vi "Describe Double Failure.vi"(1 "Expected":dbl, 2 "Got":dbl) -> (0 "Failure Description":string)   [LabVIEW 2013]
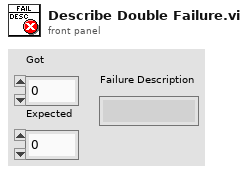
[diagram p1: front panel]
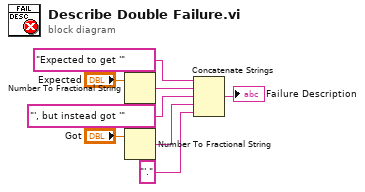
[diagram p0: block diagram]
diagram:
  n1 = Number To Fractional String(number="Expected") -> (F-format string=w4:string)  [unwired: 3 in]
  n2 = Number To Fractional String(number="Got") -> (F-format string=w7:string)  [unwired: 3 in]
  n3 = Concatenate Strings("Expected to get '", w4, "', but instead got '", w7, "'.") -> (→"Failure Description":string)
